vi "3DS Rotate Model.vi"(10 "Euler Angles":cluster{"phi":dbl, "theta":dbl, "psi":dbl}, 11 "model in":T1 {"NormalList"."z" format="%.2f"; "NormalList"."y" format="%.2f"; "NormalList"."x" format="%.2f"; "VertexList"."z" format="%.2f"; "VertexList"."y" format="%.2f"; "VertexList"."x" format="%.2f"}) -> (3 "model out":T1 {"NormalList"."z" format="%.2f"; "NormalList"."y" format="%.2f"; "NormalList"."x" format="%.2f"; "VertexList"."z" format="%.2f"; "VertexList"."y" format="%.2f"; "VertexList"."x" format="%.2f"})   [LabVIEW 2026, in "3D utilities.lvlib"]
uses:
  3D utilities.lvlib
  <vilib>/picture/3D Picture Control/Old 3D Toolkit.llb/model.ctl
  <vilib>/picture/3D Picture Control/Old 3D Toolkit.llb/point3f.ctl
  <vilib>/picture/3D Picture Control/Old 3D Toolkit.llb/VertexMode.ctl
  <vilib>/Analysis/coordinate.llb/Euler Rotation Order.ctl
  <vilib>/Analysis/coordinate.llb/3D Cartesian Coordinate Rotation (Euler) (Array).vi
  <vilib>/Analysis/NI_AALPro.lvlib
  <vilib>/picture/3D Picture Control/NI_Old 3D Toolkit.lvlib
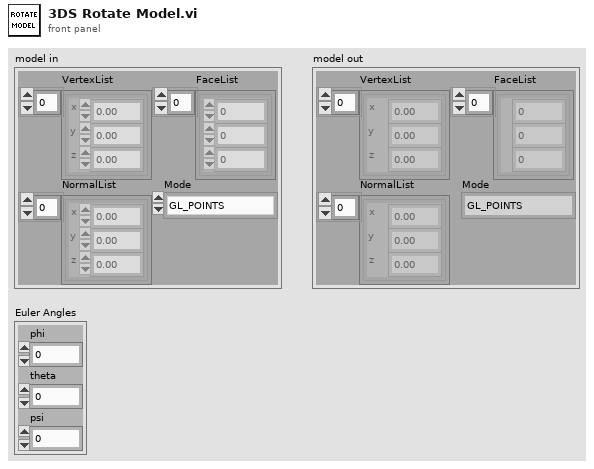
[diagram p1: front panel]
types:
  T1 = typedef "NI_3D Picture Control.lvlib/NI_Old 3D Toolkit.lvlib/model.ctl" = cluster{"VertexList":T2[], "FaceList":cluster{"v1":i32, "v2":i32, "v3":i32}[], "NormalList":T2[], "Mode":T3}
  T2 = typedef "NI_3D Picture Control.lvlib/NI_Old 3D Toolkit.lvlib/point3f.ctl" = cluster{"x":sgl, "y":sgl, "z":sgl}
  T3 = typedef "NI_3D Picture Control.lvlib/NI_Old 3D Toolkit.lvlib/VertexMode.ctl" = enum16{"GL_POINTS", "GL_LINES", "GL_LINE_LOOP", "GL_LINE_STRIP", "GL_TRIANGLES", "GL_TRIANGLE_STRIP", "GL_TRIANGLE_FAN", "GL_QUADS", "GL_QUAD_STRIP", "GL_POLYGON"}
  T4 = typedef "NI_AALPro.lvlib/Euler Rotation Order.ctl" = u16
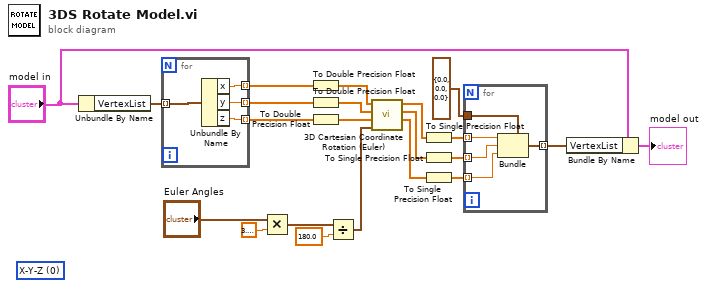
[diagram p0: block diagram]
diagram:
  (unwired) T4 0 items=["X-Y-Z", "X-Z-Y", "Y-X-Z", "Y-Z-X", "Z-X-Y", "Z-Y-X", "X-Y-X", "X-Z-X", "Y-X-Y", "Y-Z-Y", "Z-X-Z", "Z-Y-Z"] ("rotation order")
  n1 = Unbundle By Name("model in") -> ("VertexList"=w8:T2[])
  n2 = for {
    tunnel: w8 -> [w26] mode=indexing
    tunnel: [w25] -> w9 mode=indexing
    tunnel: [w24] -> w10 mode=indexing
    tunnel: [w23] -> w11 mode=indexing
    n3 = Unbundle By Name(w26) -> ("x"=w25:sgl, "y"=w24:sgl, "z"=w23:sgl)
  }
  n4 = Multiply(x="Euler Angles", y=3.141592653589793) -> (x*y=w18:cluster{"phi":dbl, "theta":dbl, "psi":dbl})
  n5 = To Double Precision Float(number=w9) -> (double precision float=w7:dbl[])
  n6 = To Double Precision Float(number=w10) -> (double precision float=w6:dbl[])
  n7 = To Double Precision Float(number=w11) -> (double precision float=w5:dbl[])
  n8 = Divide(x=w18, y=180.0) -> (x/y=w20:cluster{"phi":dbl, "theta":dbl, "psi":dbl})
  n9 = call-poly <vilib>:"3D Cartesian Coordinate Rotation (Euler).vi"("Euler Angles"=w20, "Z"=w5, "Y"=w6, "X"=w7) -> ("Z Out"=w14:dbl[], "Y Out"=w13:dbl[], "X Out"=w12:dbl[])  [unwired: 4 in, 1 out]
  n10 = To Single Precision Float(number=w12) -> (single precision float=w4:sgl[])
  n11 = To Single Precision Float(number=w13) -> (single precision float=w3:sgl[])
  n12 = To Single Precision Float(number=w14) -> (single precision float=w2:sgl[])
  n13 = for {
    tunnel: w4 -> [w31] mode=indexing
    tunnel: w3 -> [w30] mode=indexing
    tunnel: w2 -> [w29] mode=indexing
    tunnel: [w28] -> w15 mode=indexing
    tunnel: T2 {"x"=0.0, "y"=0.0, "z"=0.0} ("point3f") -> [w27]
    n14 = Bundle(cluster=w27, "x"=w31, "y"=w30, "z"=w29) -> (w28:T2)
  }
  n15 = Bundle By Name(cluster="model in", "VertexList"=w15) -> (→"model out":T1)
